vi "mocoautomation.vi"() -> (1 "Automation Settings":T1, 2 "Canceled?":bool)   [LabVIEW 2009]
panel:
  in  "Wait For Temp:":bool
  in  "Enable Temperature \nRegulation:":bool
  in  "Temperature:":dbl
  out "Interger Number of Steps?":bool
  out "Number of Steps:":dbl
  in  "Step Size:":dbl
  in  "Exposure Time:":dbl
  in  "OK Button":bool
  in  "Cancel Button":bool
  in  "Max nm":dbl
  in  "Min nm":dbl
  # "sec"
  # "nm"
  # "sec"
  # "Range:"
  # "nm to"
  # "nm"
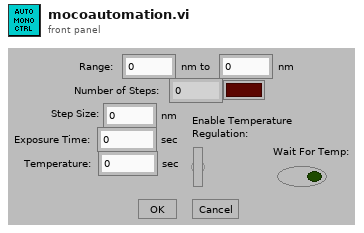
[diagram p1: front panel]
types:
  T1 = cluster{"Max nm":dbl, "Min nm":dbl, "Step Size:":dbl, "Number of Steps:":dbl, "Exposure Time:":dbl, "Regulation:":bool, "Temperature:":dbl, "Wait_For_Temp:":bool}
  T2 = cluster{"Max nm":dbl, "Min nm":dbl, "Step Size:":dbl, "Number of Steps:":dbl, "Exposure Time:":dbl, "Enable Temperature \nRegulation:":bool, "Temperature:":dbl, "Wait For Temp:":bool}
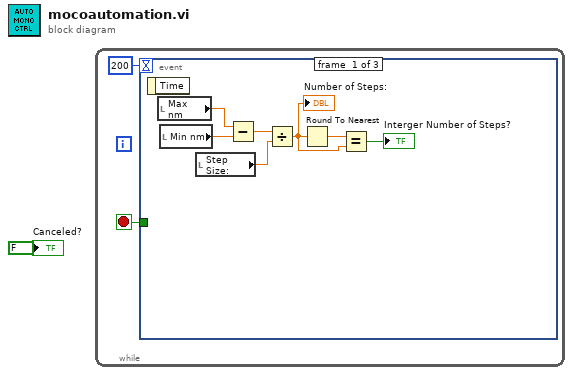
[diagram p0: block diagram]
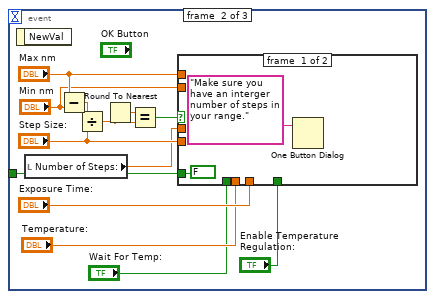
[diagram p2: hidden frame]
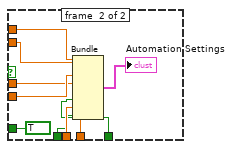
[diagram p3: hidden frame]
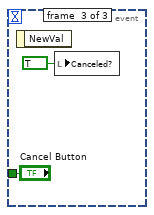
[diagram p4: hidden frame]
diagram:
  n1 = while {
    stop <- w3 stop-if-true
    n2 = event shown="[1] \"OK Button\": Value Change" {
      selector: _ -> [_ _ _]
      dyn-events: _ -> [_ _ _]
      timeout: 200 -> [_ _ _]
      tunnel: [_ w19 "Cancel Button"] -> w3
      event #0 {
        n3 = event-data() -> ()  [unwired: 1 in, 1 out]
        n4 = local read "Max nm"() -> (w8:dbl)
        n5 = local read "Min nm"() -> (w7:dbl)
        n6 = local read "Step Size:"() -> (w6:dbl)
        n7 = Subtract(x=w8, y=w7) -> (x-y=w10:dbl)
        n8 = Divide(x=w10, y=w6) -> (x/y=w5:dbl)
        "Number of Steps:" <- w5
        n9 = Round To Nearest(number=w5) -> (nearest integer value=w9:dbl)
        n10 = Equal?(x=w9, y=w5) -> (x = y?=→"Interger Number of Steps?":bool)
      }
      event #1 {
        n11 = event-data() -> ()  [unwired: 1 in, 1 out]
        n12 = local read "Number of Steps:"() -> (w15:dbl)
        n13 = Subtract(x="Max nm", y="Min nm") -> (x-y=w23:dbl)
        n14 = Divide(x=w23, y="Step Size:") -> (x/y=w20:dbl)
        n15 = Round To Nearest(number=w20) -> (nearest integer value=w21:dbl)
        n16 = Equal?(x=w21, y=w20) -> (x = y?=w22:bool)
        n17 = case shown="True" w22 {
          tunnel: [FALSE TRUE] -> w19
          tunnel: "Max nm" -> [_ w34]
          tunnel: "Min nm" -> [_ w33]
          tunnel: "Step Size:" -> [_ w32]
          tunnel: w15 -> [_ w31]
          tunnel: "Exposure Time:" -> [_ w30]
          tunnel: "Temperature:" -> [_ w28]
          tunnel: "Enable Temperature \nRegulation:" -> [_ w27]
          tunnel: "Wait For Temp:" -> [_ w26]
          frame #0 {
            n18 = One Button Dialog(message="Make sure you have an interger number of steps in your range.") -> ()  [unwired: 1 in, 1 out]
          }
          frame #1 {
            n19 = Bundle("Max nm"=w34, "Min nm"=w33, "Step Size:"=w32, "Number of Steps:"=w31, "Exposure Time:"=w30, "Enable Temperature \nRegulation:"=w27, "Temperature:"=w28, "Wait For Temp:"=w26) -> (→"Automation Settings":T2)  [unwired: 1 in]
          }
        }
      }
      event #2 {
        n20 = event-data() -> ()  [unwired: 1 in, 1 out]
        n21 = local write "Canceled?"(TRUE ("Canceled?")) -> ()
      }
    }
  }
  "Canceled?" <- FALSE ("Cancled?")
